vi "Device_GPIB_Addresses.vi"() -> (1 "HP 4275A Address":refnum<visa-resource-name>="GPIB0::3::INSTR", 2 "HP 3457A Address":refnum<visa-resource-name>="GPIB0::22::INSTR", 3 "Keithley 2400 Address":refnum<visa-resource-name>="GPIB0::24::INSTR")   [LabVIEW 2020]
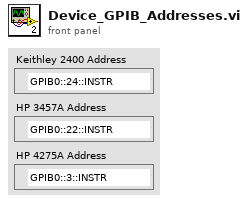
[diagram p1: front panel]
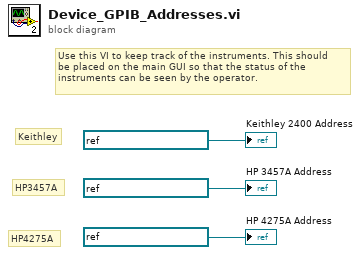
[diagram p0: block diagram]
diagram:
  # "HP4275A"
  # "HP3457A"
  # "Keithley"
  # "Use this VI to keep track of the instruments. This should\nbe placed on the main GUI so that the status of the\ninstruments can be seen by the operator."
  "HP 4275A Address" <- refnum<visa-resource-name> "GPIB0::3::INSTR" ("VISA resource name")
  "HP 3457A Address" <- refnum<visa-resource-name> "GPIB0::22::INSTR" ("VISA resource name")
  "Keithley 2400 Address" <- refnum<visa-resource-name> "GPIB0::24::INSTR" ("VISA resource name")
